vi "Torque Converter.vi"(9 "Turbine Speed (rad/s)":sgl, 10 "Impeller Speed (rad/s)":sgl) -> (1 "Turbine Torque (N-m)":sgl, 2 "Impeller Torque (N-m)":sgl)   [LabVIEW 2016, in "NI-PCG Vehicle Model.lvlib"]
uses:
  NI-PCG Vehicle Model.lvlib
  Globals/Parameters.vi
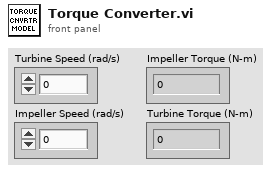
[diagram p1: front panel]
types:
  T1 = typedef "NI-PCG Vehicle Model.lvlib/Engine Parameters.ctl" = cluster{"Ambient Parameters":cluster{"Temperature (K)":sgl, "Pressure (Pa)":sgl}, "Air Parameters":cluster{"R (Ideal Gas Constant)":sgl, "Molecular Weight":sgl, "Cp (Specific Heat Constant)":sgl, "Density (kg/m^3)":sgl, "Stoichiometric A/F Ratio":sgl}, "Engine Geometry Parameters":cluster{"Cylinder Volume (l)":sgl, "J (Rotational Moment of Inertia)":sgl, "Minimuim Engine Speed":sgl, "Maximum Engine Speed":sgl, "Intake Manifold Volume (l)":sgl}, "Volumetric Efficiency Map":cluster{"MAP":sgl[], "RPM":sgl[], "Table":sgl[][]}, "Fuel LHV (J/kg)":sgl, "Combustion Efficiency Map":cluster{"Spark Timing (deg BTDC))":sgl[], "Engine Speed (RPM)":sgl[], "Combustion Efficiency":sgl[][]}, "Thermodynamic Efficiency":sgl}
  T2 = typedef "NI-PCG Vehicle Model.lvlib/Transmission Parameters.ctl" = cluster{"Final Drive Ratio":sgl, "Transmission Gear Ratios":cluster{"Gears":sgl[], "Gear Ratios":sgl[]}, "Torque Converter Map":cluster{"Speed Ratio":sgl[], "K Factor":sgl[], "Torque Ratio":sgl[]}, "Upshift Throttle":sgl[], "Downshift Throttle":sgl[], "Upshift Table":sgl[][], "Downshift Table":sgl[][], "Wait Time":u8}
  T3 = typedef "NI-PCG Vehicle Model.lvlib/Vehicle Parameters.ctl" = cluster{"Vehicle Mass (kg)":sgl, "Vehicle Cd":sgl, "Vehicle Frontal Area (m^2)":sgl, "Wheel Radius (m)":sgl, "Wheel Rolling Resistance":sgl}
  T4 = cluster{"Engine Parameters":T1, "Transmission Parameters":T2, "Vehicle Parameters":T3}
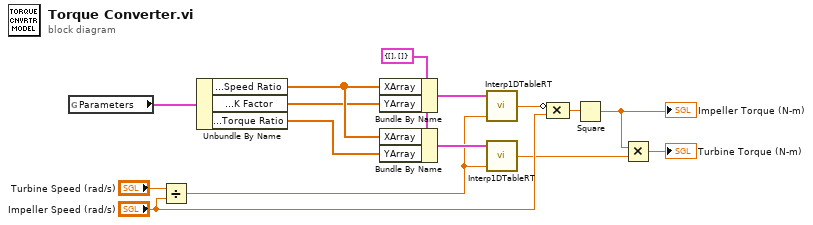
[diagram p0: block diagram]
diagram:
  w11 = cluster{"XArray":sgl[], "YArray":sgl[]} {"XArray"=[], "YArray"=[]} ("1DTable")
  n1 = global read "Parameters.vi" "Parameters"() -> (w12:T4)
  n2 = Divide(x="Turbine Speed (rad/s)", y="Impeller Speed (rad/s)") -> (x/y=w4:sgl)
  n3 = Unbundle By Name(w12) -> ("Transmission Parameters.Torque Converter Map.Speed Ratio"=w15:sgl[], "Transmission Parameters.Torque Converter Map.K Factor"=w14:sgl[], "Transmission Parameters.Torque Converter Map.Torque Ratio"=w9:sgl[])
  n4 = Bundle By Name(cluster=w11, "XArray"=w15, "YArray"=w14) -> (w10:cluster{"XArray":sgl[], "YArray":sgl[]})
  n5 = Bundle By Name(cluster=w11, "XArray"=w15, "YArray"=w9) -> (w13:cluster{"XArray":sgl[], "YArray":sgl[]})
  n6 = call <vilib>:"Interp1DTableRT.vi"("X"=w4, "1DTable"=w10) -> ("Y"=w1:sgl)  [unwired: 1 in]
  n7 = call <vilib>:"Interp1DTableRT.vi"("X"=w4, "1DTable"=w13) -> ("Y"=w3:sgl)  [unwired: 1 in]
  n8 = Compound Arithmetic op=MULTIPLY(invert w1, "Impeller Speed (rad/s)") -> (w5:sgl)
  n9 = Square(x=w5) -> (x^2=w2:sgl)
  "Impeller Torque (N-m)" <- w2
  n10 = Multiply(x=w2, y=w3) -> (x*y=→"Turbine Torque (N-m)":sgl)
